vi "ThrottleCorrection.vi"(8 "Vmin":dbl=0.075, 9 "Deadzone":dbl=0.15, 11 "Input":dbl) -> (3 "Output":dbl)   [LabVIEW 2017]
panel:
  in  "Kmax":dbl=1.4
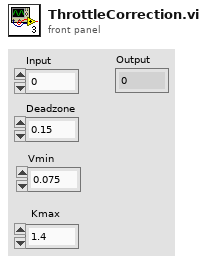
[diagram p1: front panel]
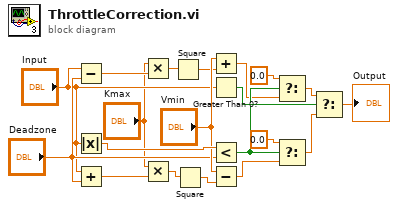
[diagram p0: block diagram]
diagram:
  n1 = Subtract(x="Input", y="Deadzone") -> (x-y=w6:dbl)
  n2 = Absolute Value(x="Input") -> (abs(x)=w19:dbl)
  n3 = Add(x="Input", y="Deadzone") -> (x+y=w7:dbl)
  n4 = Multiply(x="Kmax", y=w6) -> (x*y=w4:dbl)
  n5 = Multiply(x="Kmax", y=w7) -> (x*y=w2:dbl)
  n6 = Square(x=w4) -> (x^2=w3:dbl)
  n7 = Square(x=w2) -> (x^2=w1:dbl)
  n8 = Add(x="Vmin", y=w3) -> (x+y=w13:dbl)
  n9 = Greater Than 0?(x="Input") -> (x > 0?=w20:bool)
  n10 = Less?(x=w19, y="Deadzone") -> (x < y?=w14:bool)
  n11 = Subtract(x="Vmin", y=w1) -> (x-y=w11:dbl)
  n12 = Select(t=0.0, s=w14, f=w13) -> (s? t:f=w18:dbl)
  n13 = Select(t=0.0, s=w14, f=w11) -> (s? t:f=w16:dbl)
  n14 = Select(t=w18, s=w20, f=w16) -> (s? t:f=→"Output":dbl)
